vi "taskkill.vi"() -> ()   [LabVIEW 2015]
uses:
  kernel32.dll
panel:
  out "processID":i32
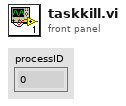
[diagram p1: front panel]
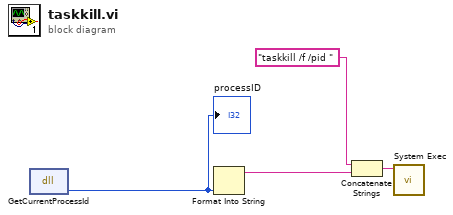
[diagram p0: block diagram]
diagram:
  n1 = dll-call lib="kernel32.dll" fn="GetCurrentProcessId"() -> ("return type"=w2:i32)  [unwired: 3 in, 2 out]
  "processID" <- w2
  n2 = Format Into String "Format Into String"(w2) -> (resulting string=w1:string)  [unwired: 3 in, 1 out]
  n3 = Concatenate Strings("taskkill /f /pid ", w1) -> (w3:string)
  n4 = call <vilib>:"System Exec.vi"("command line"=w3) -> ()  [unwired: 7 in, 4 out]
